vi "Point Number to Parametric Value.vi"(9 "Points":dbl[][](array[numeric]), 11 "Point Number":i32) -> (3 "Parametric Value":dbl)   [LabVIEW 2017]
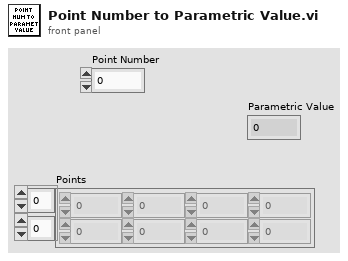
[diagram p1: front panel]
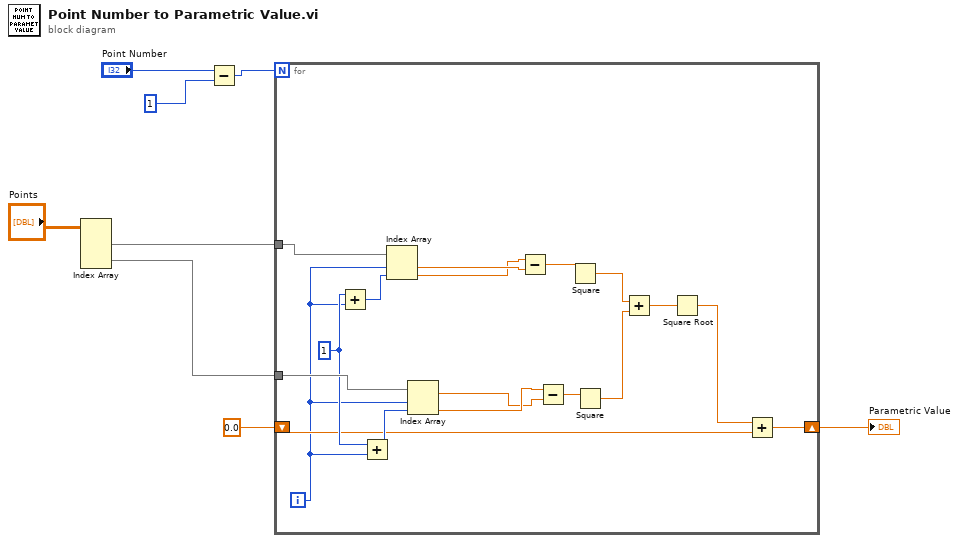
[diagram p0: block diagram]
diagram:
  n1 = Index Array(array="Points") -> (element #1=w6:dbl[], element #2=w1:dbl[])  [unwired: 4 in]
  n2 = Subtract(x="Point Number", y=1) -> (x-y=w2:i32)
  n3 = for {
    N: w2 -> [_]
    tunnel: w6 -> [w26]
    tunnel: w1 -> [w24]
    shift-right: [w9] -> w5
    shift-left: 0.0 -> [w11]
    i -> [w10]
    w22 = 1
    n4 = Add(x=w22, y=w10) -> (x+y=w25:i32)
    n5 = Add(x=w22, y=w10) -> (x+y=w23:i32)
    n6 = Index Array(array=w26, index #1=w10, index #2=w25) -> (element #1=w15:dbl, element #2=w14:dbl)
    n7 = Index Array(array=w24, index #1=w10, index #2=w23) -> (element #1=w12:dbl, element #2=w13:dbl)
    n8 = Subtract(x=w14, y=w15) -> (x-y=w18:dbl)
    n9 = Subtract(x=w13, y=w12) -> (x-y=w17:dbl)
    n10 = Square(x=w18) -> (x^2=w21:dbl)
    n11 = Square(x=w17) -> (x^2=w20:dbl)
    n12 = Add(x=w21, y=w20) -> (x+y=w19:dbl)
    n13 = Square Root(x=w19) -> (sqrt(x)=w16:dbl)
    n14 = Add(x=w16, y=w11) -> (x+y=w9:dbl)
  }
  "Parametric Value" <- w5
